vi "TSM SSC DCPower Measure.vi"(0 "DCPower TSM in":T2, 5 "Measurement Mode":T1 caption="Measurement Mode (Auto)", 11 "error in":errorcluster) -> (4 "DCPower TSM out":T2, 6 "Voltage Measurements (V)":dbl[](array[numeric]) format="%#_6p", 8 "Current Measurements (A)":dbl[](array[numeric]) format="%#_6p", 15 "error out":errorcluster)   [LabVIEW 2019]
doc: "This VI takes a Voltage and Current measurement for each session.\n\nMeasurement Mode is a recommended input. The Auto setting will check the measurement mode for each session and use the appropriate measurement method per session."
uses:
  TSM/TSM SSC DCPower.ctl
  <vilib>/NI_TestStand_SemiconductorModule/NI_TestStand_Semiconductor_Module.lvlibp/PinMap/PinQueryContext/MultiplePinMultipleSessionQueryContext/MultiplePinMultipleSessionQueryContext.lvclass
  SSC DCPower/SSC DCPower.ctl
  Shared SubVIs/TSM Pin Abstraction/TSM Pin Information.ctl
  Shared SubVIs/TSM Pin Abstraction/TSM Pin Type Identifier.ctl
  Shared SubVIs/TSM Pin Abstraction/TSM Expanded Pin Information.ctl
  SSC DCPower/Measure/SSC DCPower Measurement Mode.ctl
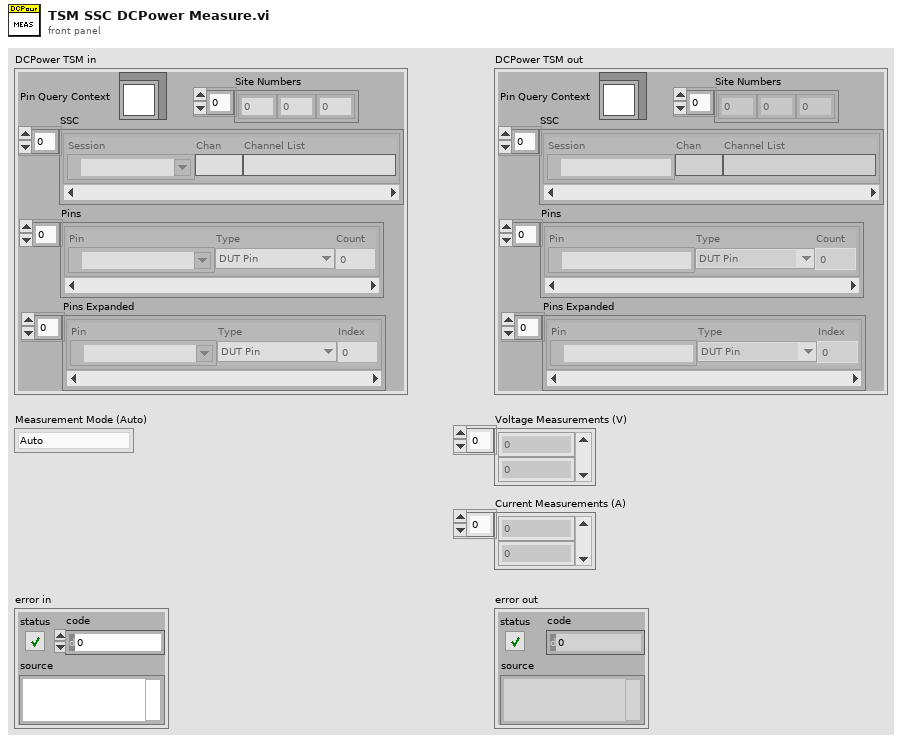
[diagram p1: front panel]
types:
  T1 = typedef "SSC DCPower Measurement Mode.ctl" = enum16{"Auto", "Measure Multiple", "Software Triggers"}
  T2 = typedef "TSM SSC DCPower.ctl" = cluster{"Pin Query Context":refnum<class "MultiplePinMultipleSessionQueryContext.lvclass">, "SSC":T3[], "Site Numbers":i32[], "Pins":T4[], "Pins Expanded":T6[]}
  T3 = typedef "SSC DCPower.ctl" = cluster{"Session":refnum<k15>, "Chan":string, "Channel List":string}
  T4 = typedef "TSM Pin Information.ctl" = cluster{"Pin":tag, "Type":T5, "Count":i32}
  T5 = typedef "TSM Pin Type Identifier.ctl" = enum8{"DUT Pin", "System Pin", "Pin Group", "Not Determined"}
  T6 = typedef "TSM Expanded Pin Information.ctl" = cluster{"Pin":tag, "Type":T5, "Index":i32}
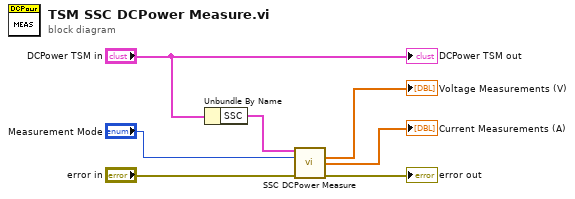
[diagram p0: block diagram]
diagram:
  n1 = Unbundle By Name("DCPower TSM in") -> ("SSC"=w4:T3[])
  n2 = call "SSC DCPower Measure.vi"("DCPower SSC in"=w4, "Measurement Mode"="Measurement Mode", "error in"="error in") -> ("Voltage Measurements (V)"=→"Voltage Measurements (V)":dbl[], "Current Measurements (A)"=→"Current Measurements (A)":dbl[], "error out"=→"error out":errorcluster)  [unwired: 9 in, 1 out]
  "DCPower TSM out" <- "DCPower TSM in"
